vi "initStateToState0.vi"(8 "error in (no error)":errorcluster, 11 "OptCtrl in":refnum<class "OptCtrl.lvclass">) -> (0 "error out":errorcluster, 3 "OptCtrl out":refnum<class "OptCtrl.lvclass">)   [LabVIEW 2016, in "OptCtrl.lvclass"]
doc: "Initialize the state to the state 0 in the basis of degree of freedom."
uses:
  OptCtrl.lvclass
  OptCtrl.lvclass/OptCtrl.ctl
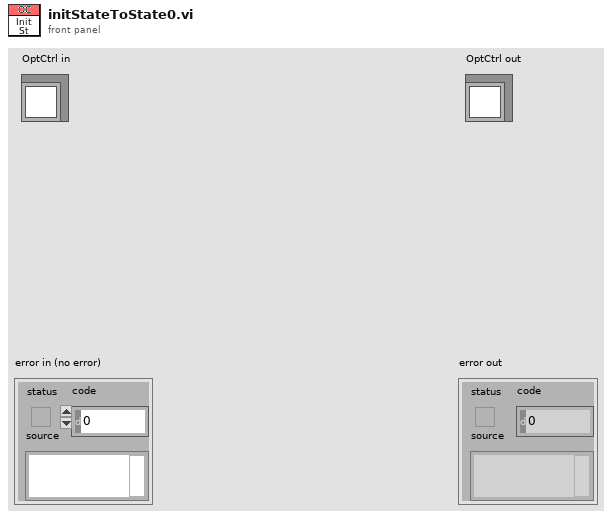
[diagram p1: front panel]
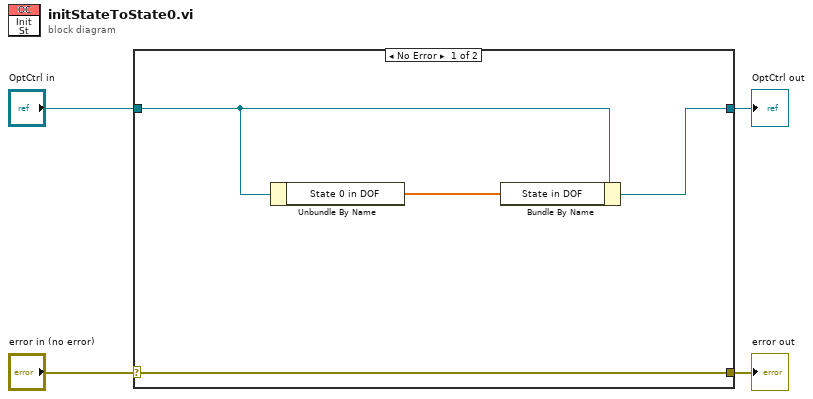
[diagram p0: block diagram]
diagram:
  n1 = case shown="No Error" "error in (no error)" {
    selector: "error in (no error)" -> [w8 w10]
    tunnel: [w8 w10] -> w3
    tunnel: [w7 w9] -> w1
    tunnel: "OptCtrl in" -> [w6 w9]
    frame No Error {
      n2 = Unbundle By Name(w6) -> ("State 0 in DOF"=w5:dbl[])
      n3 = Bundle By Name(cluster=w6, "State in DOF"=w5) -> (w7:refnum<class "OptCtrl.lvclass">)
    }
    frame Error {
    }
  }
  "error out" <- w3
  "OptCtrl out" <- w1
